vi "Pulse Delay Test.vi"() -> ()   [LabVIEW 2012]
panel:
  in  "Delay step width":dbl
  in  "APD signal width":dbl
  out "Array":T1(array[cluster])
  in  "Tracking Interval":dbl
  in  "file path":path
  in  "Path to spinapi.dll":path=path "C:/SpinCore/SpinAPI/dll/spinapi64.dll"
  in  "Delay Max":dbl
  in  "Delay min":dbl
  in  "AOM Pulse length":dbl=3e-07
  in  "Sig/Ref pause":dbl
  in  "AOM Rest time":dbl
  in  "N Loop":i32=25000
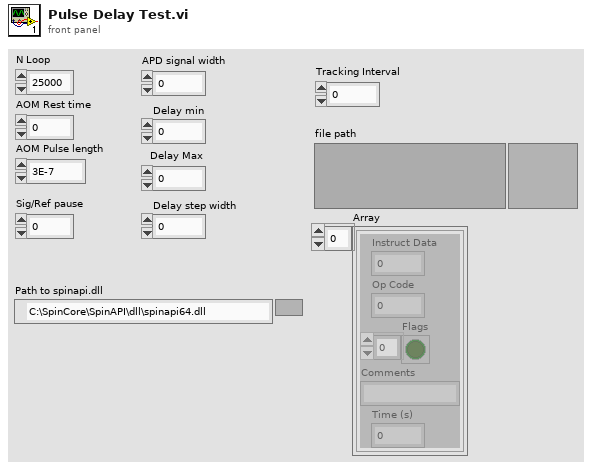
[diagram p1: front panel]
types:
  T1 = cluster{"Instruct Data":i32, "Op Code":i32, "Flags":bool[], "Comments":string, "Time (s)":dbl}[]
  T2 = enum16{"Pulse Program", "Frequency Registers", "TX Phase Registers", "RX Phase Registers"}
  T3 = cluster{"Instruct Data":i32, "Op Code":i32, "Flags":bool[], "Comments":string, "Time (s)":dbl}
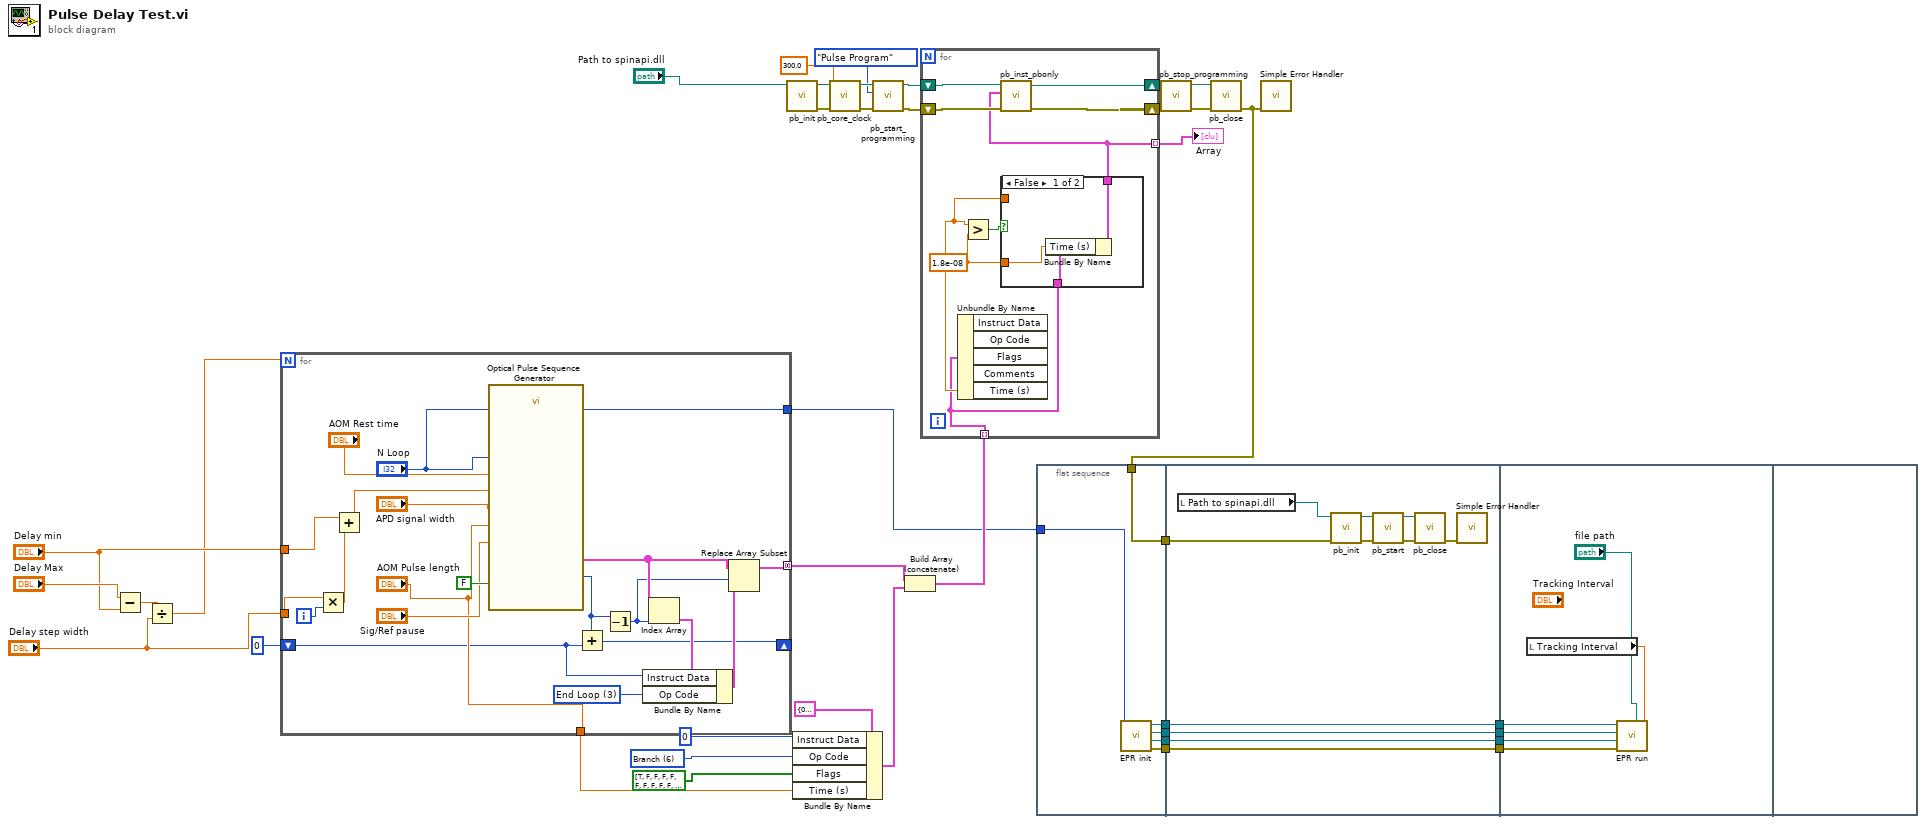
[diagram p0: block diagram]
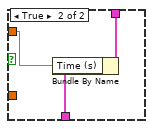
[diagram p2: hidden frame]
diagram:
  w34 = 6 items=["Continue", "Stop", "Loop", "End Loop", "JSR", "RTS", "Branch", "Long Delay", "Wait"] ("Op Code")
  n1 = Subtract(x="Delay Max", y="Delay min") -> (x-y=w37:dbl)
  n2 = Divide(x=w37, y="Delay step width") -> (x/y=w7:dbl)
  n3 = for {
    N: w7 -> [_]
    tunnel: "Delay min" -> [w54]
    tunnel: [w45] -> w2 mode=concatenating
    tunnel: ["AOM Pulse length"] -> w32
    tunnel: ["N Loop"] -> w8
    tunnel: "Delay step width" -> [w41]
    shift-right: [w43] -> _
    shift-left: 0 -> [w44]
    i -> [w56]
    w49 = 3 items=["Continue", "Stop", "Loop", "End Loop", "JSR", "RTS", "Branch", "Long Delay", "Wait"] ("Op Code")
    n4 = Multiply(x=w41, y=w56) -> (x*y=w55:dbl)
    n5 = Add(x=w54, y=w55) -> (x+y=w53:dbl)
    n6 = call "Optical Pulse Sequence Generator.vi"("ref?"=FALSE, "N Loop"="N Loop", "Sig/Ref pause"="Sig/Ref pause", "AOM Rest time"="AOM Rest time", "Signal delay"=w53, "APD signal width"="APD signal width", "AOM Pulse length"="AOM Pulse length") -> ("Array"=w48:T1, "No. Instructions"=w42:i32)  [unwired: 3 in]
    n7 = Add(x=w42, y=w44) -> (x+y=w43:i32)
    n8 = Decrement(x=w42) -> (x-1=w47:i32)
    n9 = Index Array(array=w48, index=w47) -> (element=w50:T3)
    n10 = Bundle By Name(cluster=w50, "Instruct Data"=w44, "Op Code"=w49) -> (w46:T3)
    n11 = Replace Array Subset(array=w48, new element=w46, index=w47) -> (w45:T1)
  }
  n12 = call "pb_init.vi"("path in"="Path to spinapi.dll") -> ("error out"=w23:errorcluster, "path out"=w21:path)  [unwired: 3 in, 6 out]
  n13 = Bundle By Name(cluster=T3 {"Instruct Data"=0, "Op Code"=0, "Flags"=[FALSE, FALSE, FALSE, FALSE, FALSE, FALSE, FALSE, FALSE, FALSE, FALSE, FALSE, FALSE, FALSE, FALSE, FALSE, FALSE, FALSE, FALSE, FALSE, FALSE, FALSE, TRUE, TRUE, TRUE], "Comments"="", "Time (s)"=0.01} ("PB Inst 2"), "Instruct Data"=0, "Op Code"=w34, "Flags"=bool[] [TRUE, FALSE, FALSE, FALSE, FALSE, FALSE, FALSE, FALSE, FALSE, FALSE, FALSE, FALSE, FALSE, FALSE, FALSE, FALSE, FALSE, FALSE, FALSE, FALSE, FALSE, TRUE, TRUE, TRUE], "Time (s)"=w32) -> (w31:T3)
  n14 = call "pb_core_clock.vi"("error in (no error)"=w23, "clock_freq (MHz)"=300.0, "path in"=w21) -> ("error out"=w24:errorcluster, "path out"=w22:path)  [unwired: 7 in]
  n15 = call "pb_start_programming.vi"("error in (no error)"=w24, "Device"=T2."Pulse Program", "path in"=w22) -> ("error out"=w27:errorcluster, "path out"=w26:path)  [unwired: 1 in, 6 out]
  n16 = Build Array (concatenate)(w2, w31) -> (w17:T1)
  n17 = for {
    shift-right: [w66] -> w28
    shift-left: w26 -> [w68]
    shift-right: [w65] -> w29
    shift-left: w27 -> [w67]
    tunnel: w17 -> [w61] mode=indexing
    tunnel: [w60] -> w4 mode=indexing
    w63 = 1.8e-08 ("y")
    n18 = Unbundle By Name(w61) -> ("Time (s)"=w62:dbl)  [unwired: 4 out]
    n19 = Greater?(x=w62, y=w63) -> (0:w64:bool)
    n20 = case shown="False" w64 {
      tunnel: w63 -> [w70 _]
      tunnel: w62 -> [_ w74]
      tunnel: w61 -> [w71 w73]
      tunnel: [w69 w72] -> w60
      frame False {
        n21 = Bundle By Name(cluster=w71, "Time (s)"=w70) -> (w69:T3)
      }
      frame True {
        n22 = Bundle By Name(cluster=w73, "Time (s)"=w74) -> (w72:T3)
      }
    }
    n23 = call "pb_inst_pbonly.vi"("error in (no error)"=w67, "PB Instruction"=w60, "path in"=w68) -> ("error out"=w65:errorcluster, "path out"=w66:path)  [unwired: 2 in, 5 out]
  }
  "Array" <- w4
  n24 = flat-sequence {
    tunnel: [w80] -> w16
    tunnel: [w79] -> w15
    tunnel: [w78] -> w14
    tunnel: [w77] -> w13
    tunnel: w8 -> [w76]
    tunnel: w6 -> [w75]
    tunnel: [w75] -> w5
    tunnel: [w85] -> w12
    tunnel: w16 -> [w85]
    tunnel: [w84] -> w11
    tunnel: w15 -> [w84]
    tunnel: [w83] -> w10
    tunnel: w14 -> [w83]
    tunnel: [w82] -> w9
    tunnel: w13 -> [w82]
    tunnel: w5 -> [w81]
    tunnel: w12 -> [w96]
    tunnel: w11 -> [w95]
    tunnel: w10 -> [w94]
    tunnel: w9 -> [w93]
    frame #0 {
      n25 = call "EPR init.vi"("N loops"=w76) -> ("error out"=w77:errorcluster, "ref task out"=w78:refnum<k21>, "sig task out"=w79:refnum<k21>, "clock task out"=w80:refnum<k21>)  [unwired: 7 in]
    }
    frame #1 {
      n26 = local read "Path to spinapi.dll"() -> (w91:path)
      n27 = call "pb_init.vi"("error in (no error)"=w81, "path in"=w91) -> ("error out"=w88:errorcluster, "path out"=w87:path)  [unwired: 1 in, 7 out]
      n28 = call "pb_start.vi"("error in (no error)"=w88, "path in"=w87) -> ("error out"=w89:errorcluster, "path out"=w86:path)  [unwired: 1 in, 7 out]
      n29 = call "pb_close.vi"("error in (no error)"=w89, "path in"=w86) -> ("error out"=w90:errorcluster)  [unwired: 9 out]
      n30 = call <vilib>:"Simple Error Handler.vi"("error in (no error)"=w90) -> ()  [unwired: 1 in, 8 out]
    }
    frame #2 {
      n31 = local read "Tracking Interval"() -> (w97:dbl)
      n32 = call "EPR run.vi"("control task in"=w96, "sig task in"=w95, "ref task in"=w94, "error in"=w93, "file path (dialog if empty)"="file path", "Measurement Interval"=w97) -> ()  [unwired: 4 in]
    }
    frame #3 {
    }
  }
  n33 = call "pb_stop_programming.vi"("error in (no error)"=w29, "path in"=w28) -> ("error out"=w20:errorcluster, "path out"=w19:path)  [unwired: 1 in, 7 out]
  n34 = call "pb_close.vi"("error in (no error)"=w20, "path in"=w19) -> ("error out"=w6:errorcluster)  [unwired: 9 out]
  n35 = call <vilib>:"Simple Error Handler.vi"("error in (no error)"=w6) -> ()  [unwired: 1 in, 8 out]
